vi "Get All Headers.vi"(8 "error in (no error)":errorcluster, 11 "Response Headers in":refnum<class "Response Headers.lvclass">) -> (0 "error out":errorcluster, 1 "Values":string[](array[string]), 2 "Names":string[](array[string]), 3 "Response Headers out":refnum<class "Response Headers.lvclass">)   [LabVIEW 2018, in "REST Client_JKI.lvlib" / "Response Headers.lvclass"]
doc: "Get all HTTP response hader names and corresponding values."
uses:
  Response Headers.lvclass
  Response Headers.lvclass/Response Headers.ctl
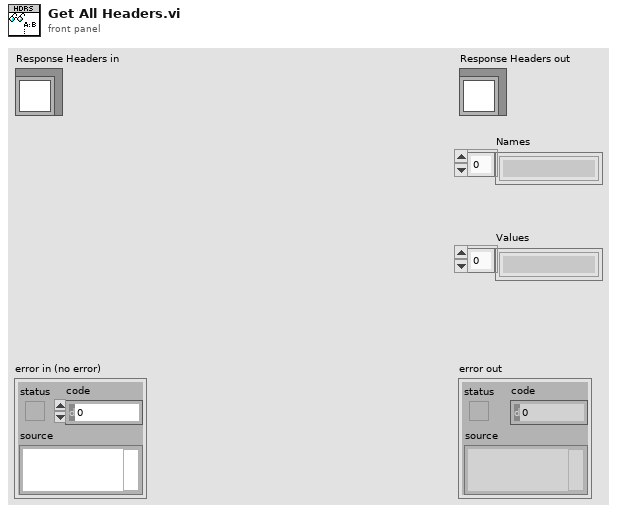
[diagram p1: front panel]
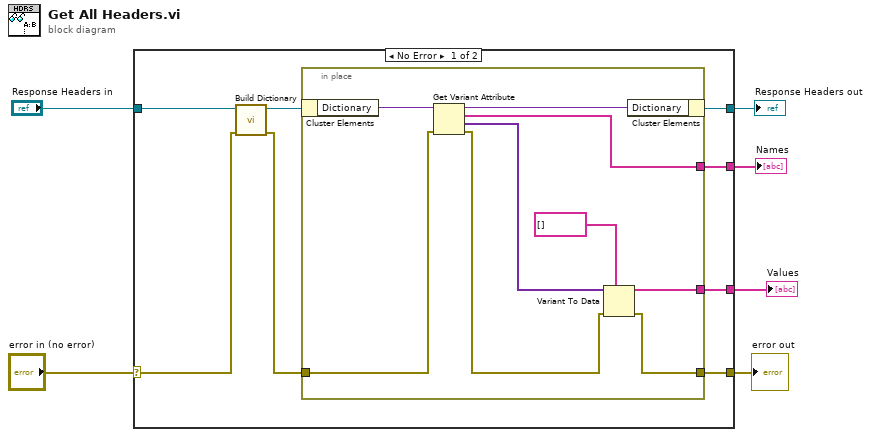
[diagram p0: block diagram]
diagram:
  n1 = case shown="No Error" "error in (no error)" {
    selector: "error in (no error)" -> [w10 w25]
    tunnel: [w13 w25] -> w5
    tunnel: [w14 w24] -> w3
    tunnel: "Response Headers in" -> [w12 w24]
    tunnel: [w8 _] -> w2
    tunnel: [w7 _] -> w1
    frame No Error {
      n2 = call "Build Dictionary.vi"("error in (no error)"=w10, "Response Headers in"=w12) -> ("error out"=w9:errorcluster, "Response Headers out"=w11:refnum<class "Response Headers.lvclass">)  [unwired: 8 in]
      n3 = in-place {
        in-place-border: w9 -> [w21]
        in-place-border: [w16] -> w13
        in-place-border: [w20] -> w8
        in-place-border: [w15] -> w7
        n4 = in-place-cluster #1(w11) -> ("Dictionary"=w23:variant)
        n5 = Get Variant Attribute(Variant=w23, error in=w21) -> (duplicate Variant=w22:variant, names=w20:string[], values=w19:variant[], error out=w17:errorcluster)  [unwired: 2 in]
        n6 = Variant To Data(error in=w17, type=string[] [] ("Names"), Variant=w19) -> (data=w15:string[], error out=w16:errorcluster)
        n7 = in-place-cluster #1("Dictionary"=w22) -> (w14:refnum<class "Response Headers.lvclass">)
      }
    }
    frame Error {
    }
  }
  "error out" <- w5
  "Response Headers out" <- w3
  "Names" <- w2
  "Values" <- w1
